vi "Autonomous.vi"   [LabVIEW 2020]
doc: "This VI starts when autonomous period begins, and will automatically be terminated when it ends. You can carry out timed or sensor driven operations directly to I/O or to subsystems without needing to return to the caller."
uses:
  Framework/Robot Global Data.vi
  <vilib>/Rock Robotics/Network Tables/NT Read Number.vi
  <vilib>/Rock Robotics/Network Tables/NT Read String.vi
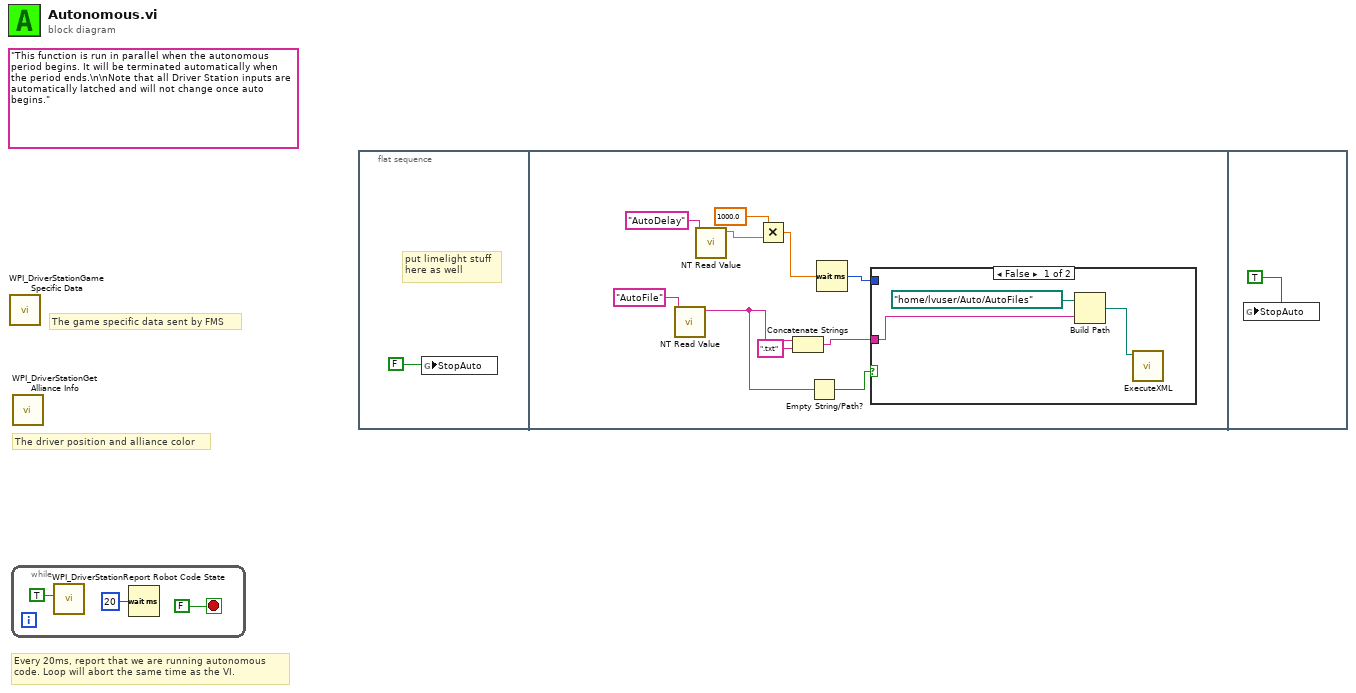
[diagram p0: block diagram]
diagram:
  (unwired) "This function is run in parallel when the autonomous period begins. It will be terminated automatically when the period ends.\n\nNote that all Driver Station inputs are automatically latched and will not change once auto begins."
  # "The game specific data sent by FMS"
  # "Every 20ms, report that we are running autonomous\ncode. Loop will abort the same time as the VI."
  # "The driver position and alliance color"
  n1 = call <vilib>:"WPI_DriverStationGame Specific Data.vi"() -> ()  [unwired: 11 in, 1 out]
  n2 = while {
    stop <- FALSE stop-if-true
    n3 = call <vilib>:"WPI_DriverStationReport Robot Code State.vi"("Autonomous"=TRUE) -> ()  [unwired: 10 in, 1 out]
    n4 = Wait (ms)(milliseconds to wait=u32 20) -> ()  [unwired: 1 out]
  }
  n5 = call <vilib>:"WPI_DriverStationGet Alliance Info.vi"() -> ()  [unwired: 12 out]
  n6 = flat-sequence {
    frame #0 {
      # "put limelight stuff\nhere as well"
      n7 = global write "Robot Global Data.vi" "StopAuto"(FALSE) -> ()
    }
    frame #1 {
      n8 = call-poly <vilib>:"NT Read Value.vi"("Name"="AutoFile") -> ("String"=w6:string)  [unwired: 9 in, 1 out]
      n9 = call-poly <vilib>:"NT Read Value.vi"("Name"="AutoDelay") -> ("Numeric"=w13:dbl)  [unwired: 9 in, 1 out]
      n10 = Multiply(x=1000.0, y=w13) -> (x*y=w10:dbl)
      n11 = Concatenate Strings(w6, ".txt" ("string")) -> (w7:string)
      n12 = Empty String/Path?(string/path=w6) -> (empty?=w5:bool)
      n13 = Wait (ms)(milliseconds to wait=w10) -> (millisecond timer value=w11:u32)
      n14 = case shown="False" w5 {
        tunnel: w11 -> [_ _]
        tunnel: w7 -> [w15 _]
        frame False {
          n15 = Build Path(base path=path "/home/lvuser/Auto/AutoFiles", name or relative path=w15) -> (appended path=w16:path)
          n16 = call "ExecuteXML.vi"("Auto File Path"=w16) -> ()  [unwired: 10 in, 1 out]
        }
        frame True {
        }
      }
    }
    frame #2 {
      n17 = global write "Robot Global Data.vi" "StopAuto"(TRUE) -> ()
    }
  }
